vi "peek_address.vi"(6 "timeout (25000ms)":i32=25000, 8 "error in (no error)":errorcluster, 9 "bytes":i32, 10 "address":i32, 11 "daemon reference in":refnum<k5>) -> (0 "error out":errorcluster, 2 "value":i32, 3 "daemon reference out":refnum<k5>, 5 "command out":string="random")   [LabVIEW 2017]
doc: "<b>Command: </b>\"peek_address\"\n\n<b>Description: </b>This command peeks at a variable stored in memory on the target using an address input.\n\n<b>Parameters: </b> \n\n 1. Address of Variable\n 2. Bytes to read\n\n<b>Note: </b>This command will only work on DEV builds of the target and as long as the relevant firmware json file has been loaded using \"load_firmware_json\" command.\n____________________________________________\nDIPC 692 Daemon API 10.0.0.1\nSam Tee - Dyson Technology Ltd\nCopyright (c) 2024, Dyson Technology Ltd"
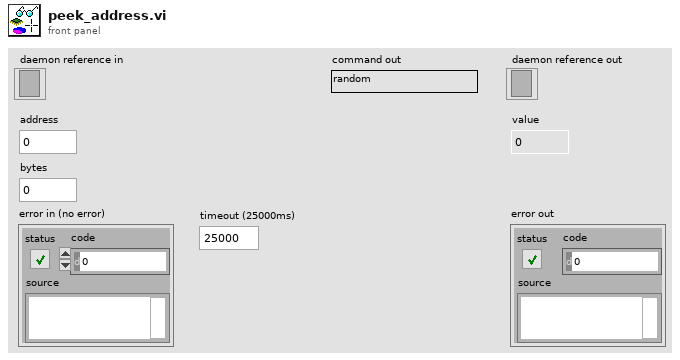
[diagram p1: front panel]
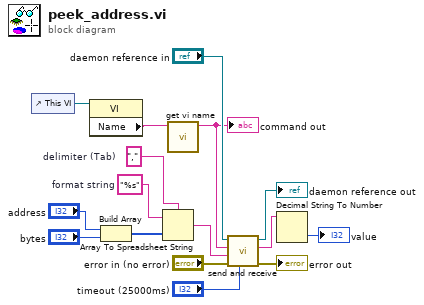
[diagram p0: block diagram]
diagram:
  w8 = ","  # delimiter (Tab)
  w7 = "%s"  # format string
  n1 = control-ref of="This VI"() -> (w11:refnum<vi>)
  n2 = property class="VI"(reference=w11) -> ("Name"=w10:string)  [unwired: 1 in, 2 out]
  n3 = Build Array("address", "bytes") -> (w6:i32[])
  n4 = Array To Spreadsheet String(delimiter (Tab)=w8, array=w6, 3:w7) -> (spreadsheet string=w3:string)
  n5 = call "get vi name.vi"("library.lvlib:name.vi"=w10) -> ("vi name"=w9:string)  [unwired: 10 in]
  "command out" <- w9
  n6 = call "send and receive.vi"("timeout (25000ms)"="timeout (25000ms)", "error in (no error)"="error in (no error)", "data"=w3, "command"=w9, "daemon reference in"="daemon reference in") -> ("error out"=→"error out":errorcluster, "response"=w2:string, "daemon reference out"=→"daemon reference out":refnum<k5>)  [unwired: 4 in]
  n7 = Decimal String To Number(string=w2) -> (number=→"value":i32)  [unwired: 2 in, 1 out]
